vi "StopCCLM.vi"(0 "VISA Resource Name":refnum<visa-resource-name>="COM1", 5 "Stop Stimulation":bool, 11 "error in (no error)":errorcluster) -> (4 "VISA resource name out":refnum<visa-resource-name>, 8 "Stimulation Stopped":bool, 15 "error out":errorcluster)   [LabVIEW 2020]
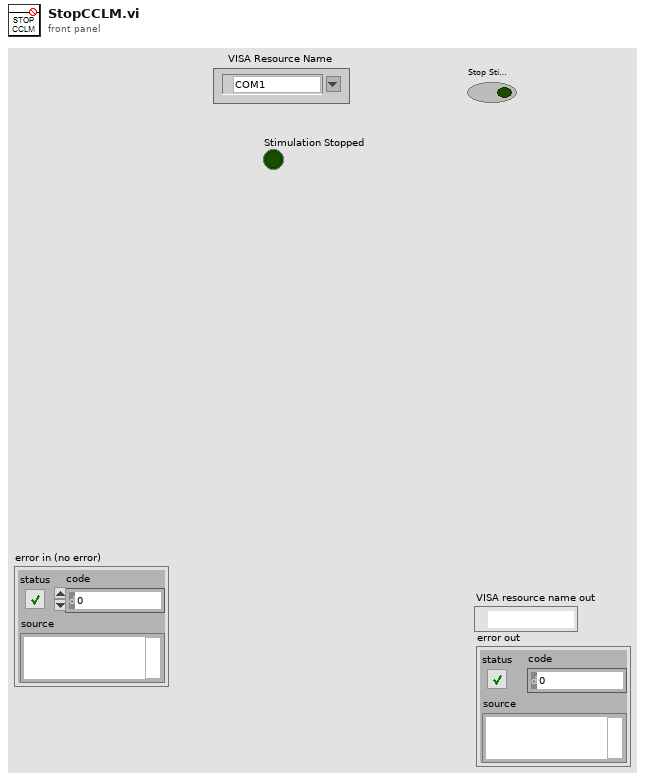
[diagram p1: front panel]
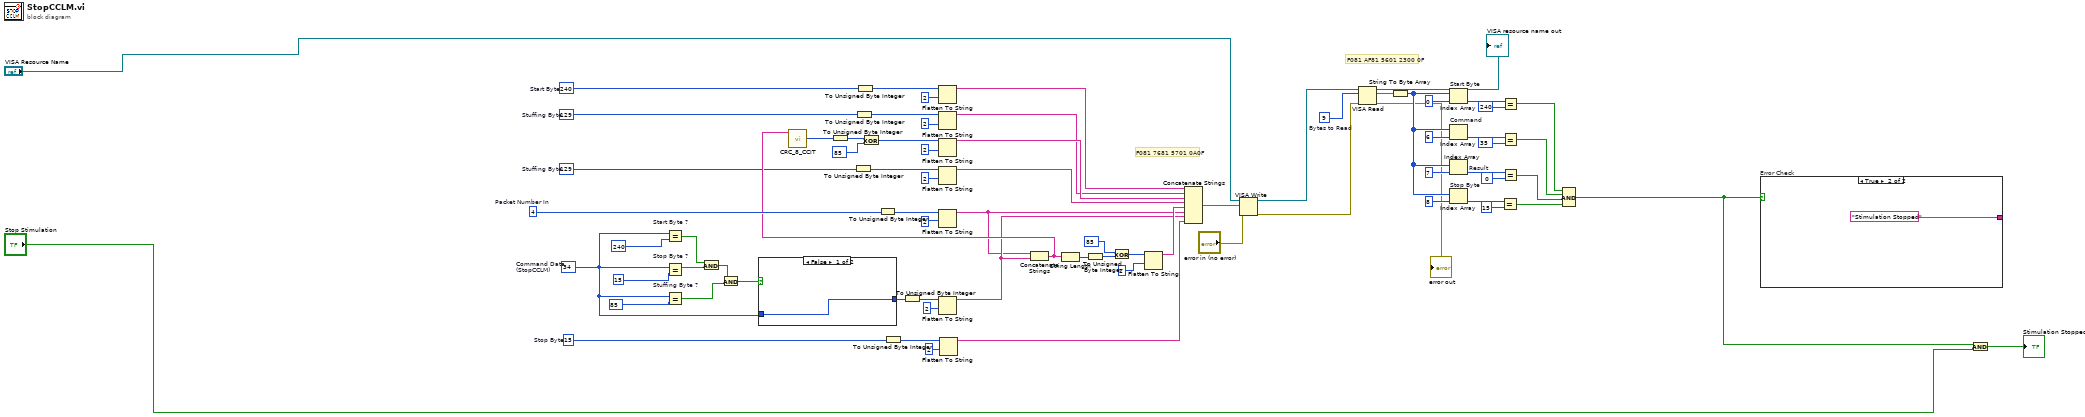
[diagram p0: block diagram]
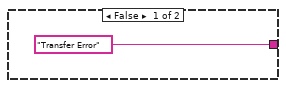
[diagram p2: hidden frame]
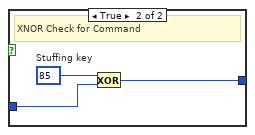
[diagram p3: hidden frame]
diagram:
  w75 = u8 4  # Packet Number In
  w19 = 9  # Bytes to Read
  w38 = 15  # Stop Byte
  w41 = 129  # Stuffing Byte
  w42 = 129  # Stuffing Byte
  w40 = 240  # Start Byte
  w56 = 34  # Command Data (StopCCLM)
  # "F081 7681 5701 0A0F"
  # "F081 AF81 5601 2300 0F"
  n1 = Equal? "Start Byte ?"(x=w56, y=240 ("IntAck")) -> (x = y?=w29:bool)
  n2 = Equal? "Stop Byte ?"(x=w56, y=15 ("IntAck")) -> (x = y?=w30:bool)
  n3 = Equal? "Stuffing Byte ?"(x=w56, y=85 ("IntAck")) -> (x = y?=w32:bool)
  n4 = And(x=w29, y=w30) -> (x .and. y?=w31:bool)
  n5 = And(x=w31, y=w32) -> (x .and. y?=w33:bool)
  n6 = case shown="False" w33 {
    tunnel: w56 -> [w76 w79]
    tunnel: [w76 w77] -> w57
    frame False {
    }
    frame True {
      w78 = 85  # Stuffing key
      # "XNOR Check for Command"
      n7 = Exclusive Or(1:w79, 2:w78) -> (0:w77:i32)
    }
  }
  n8 = To Unsigned Byte Integer(number=w42) -> (unsigned 8bit integer=w45:u8)
  n9 = To Unsigned Byte Integer(number=w41) -> (unsigned 8bit integer=w44:u8)
  n10 = To Unsigned Byte Integer(number=w40) -> (unsigned 8bit integer=w43:u8)
  n11 = To Unsigned Byte Integer(number=w75) -> (unsigned 8bit integer=w64:u8)
  n12 = To Unsigned Byte Integer(number=w38) -> (unsigned 8bit integer=w39:u8)
  n13 = To Unsigned Byte Integer(number=w57) -> (unsigned 8bit integer=w63:u8)
  n14 = Flatten To String(anything=w43, byte order (0:big-endian, network order)=2) -> (data string=w34:string)  [unwired: 2 in, 2 out]
  n15 = Flatten To String(anything=w44, byte order (0:big-endian, network order)=2) -> (data string=w35:string)  [unwired: 2 in, 2 out]
  n16 = Flatten To String(anything=w45, byte order (0:big-endian, network order)=2) -> (data string=w37:string)  [unwired: 2 in, 2 out]
  n17 = Flatten To String(anything=w64, byte order (0:big-endian, network order)=2) -> (data string=w58:string)  [unwired: 2 in, 2 out]
  n18 = Flatten To String(anything=w63, byte order (0:big-endian, network order)=2) -> (data string=w59:string)  [unwired: 2 in, 2 out]
  n19 = Flatten To String(anything=w39, byte order (0:big-endian, network order)=2) -> (data string=w28:string)  [unwired: 2 in, 2 out]
  n20 = Concatenate Strings(w58, w59) -> (w66:string)
  n21 = call "CRC_8_CCIT.vi"("Data String"=w66) -> ("Numeric"=w65:u8)  [unwired: 10 in]
  n22 = To Unsigned Byte Integer(number=w65) -> (unsigned 8bit integer=w68:u8)
  n23 = Exclusive Or(1:u8 85, 2:w68) -> (0:w67:u8)
  n24 = Flatten To String(anything=w67, byte order (0:big-endian, network order)=2) -> (data string=w36:string)  [unwired: 2 in, 2 out]
  n25 = String Length(string=w66) -> (length=w61:i32)
  n26 = To Unsigned Byte Integer(number=w61) -> (unsigned 8bit integer=w71:u8)
  n27 = Exclusive Or(1:w71, 2:u8 85) -> (0:w70:u8)
  n28 = Flatten To String(anything=w70, byte order (0:big-endian, network order)=2) -> (data string=w62:string)  [unwired: 2 in, 2 out]
  n29 = Concatenate Strings(w34, w35, w36, w37, w62, w58, w59, w28) -> (w27:string)
  n30 = VISA Write(VISA resource name="VISA Resource Name", write buffer=w27, error in (no error)="error in (no error)") -> (VISA resource name out=w8:refnum<visa-resource-name>, error out=w7:errorcluster)  [unwired: 1 out]
  n31 = VISA Read(VISA resource name=w8, byte count=w19, error in (no error)=w7) -> (VISA resource name out=→"VISA resource name out":refnum<visa-resource-name>, read buffer=w4:string, error out=→"error out":errorcluster)  [unwired: 1 out]
  n32 = String To Byte Array(string=w4) -> (unsigned byte array=w10:u8[])
  n33 = Index Array "Start Byte"(array=w10, index=0) -> (element=w22:u8)
  n34 = Index Array "Command"(array=w10, index=6) -> (element=w20:u8)
  n35 = Index Array "Result"(array=w10, index=7) -> (element=w9:u8)
  n36 = Index Array "Stop Byte"(array=w10, index=8) -> (element=w16:u8)
  n37 = Equal?(x=w16, y=u16 15) -> (x = y?=w11:bool)
  n38 = Equal?(x=w22, y=u16 240) -> (x = y?=w12:bool)
  n39 = Equal?(x=w20, y=u16 35) -> (x = y?=w13:bool)
  n40 = Equal?(x=w9, y=u16 0) -> (x = y?=w14:bool)
  n41 = Compound Arithmetic op=AND(w12, w13, w14, w11) -> (w6:bool)
  n42 = case "Error Check" shown="True" w6 {
    tunnel: ["Transfer Error" "Stimulation Stopped"] -> _
    frame False {
    }
    frame True {
    }
  }
  n43 = And(x=w6, y="Stop Stimulation") -> (x .and. y?=→"Stimulation Stopped":bool)
